vi "etc_XCITE_ExecuteCommand.vi"(8 "error in (no error)":errorcluster {"code" format="%x"}, 10 "command":string, 11 "h":u64) -> (0 "error out":errorcluster {"code" format="%x"}, 1 "answer":string, 2 "ErrorMessage":i32 format="%x", 3 "h out":u64)   [LabVIEW 2019, in "XCite.lvlib"]
doc: "Sends a command to execute on the slelected X-cite device."
uses:
  XCite.lvlib
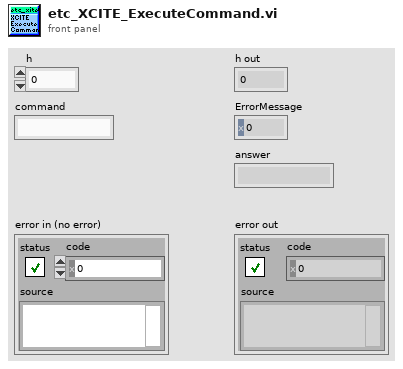
[diagram p1: front panel]
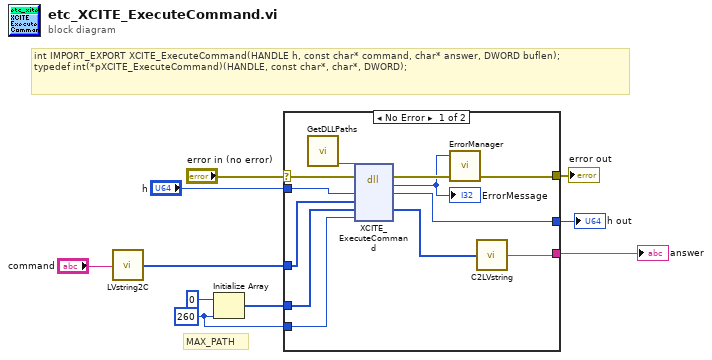
[diagram p0: block diagram]
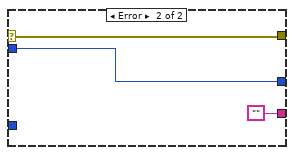
[diagram p2: hidden frame]
diagram:
  w3 = u16 260 ("dimension size")
  # "MAX_PATH"
  # "int IMPORT_EXPORT XCITE_ExecuteCommand(HANDLE h, const char* command, char* answer, DWORD buflen);\ntypedef int(*pXCITE_ExecuteCommand)(HANDLE, const char*, char*, DWORD);"
  n1 = call "LVstring2C.vi"("LVString"="command") -> ("CString"=w1:u8[])  [unwired: 3 in, 1 out]
  n2 = Initialize Array(u8 0, w3) -> (w4:u8[])
  n3 = case shown="No Error" "error in (no error)" {
    selector: "error in (no error)" -> [w22 w25]
    tunnel: [w20 w25] -> w10
    tunnel: "h" -> [w18 w24]
    tunnel: [w17 w24] -> w8
    tunnel: [w11 ""] -> w6
    tunnel: w1 -> [w15 _]
    tunnel: w4 -> [w14 _]
    tunnel: w3 -> [w13 _]
    frame No Error {
      n4 = call "GetDLLPaths.vi"() -> ("etc_xcite_path"=w16:path)  [unwired: 8 in, 3 out]
      n5 = dll-call lib="C:/LabVIEWDevFall2024/pco.labview/labview_sdk/runtime/bin64/etc_xcite.dll" fn="XCITE_ExecuteCommand"(path in=w16, error in=w22, "h"=w18, "command"=w15, "answer"=w14, "buflen"=w13) -> (error out=w21:errorcluster, "return type"=w19:i32, "h"=w17:u64, "answer"=w12:u8[])  [unwired: 3 in, 1 out]
      "ErrorMessage" <- w19
      n6 = call "ErrorManager.vi"("error in (no error)"=w21, "error code"=w19) -> ("error out"=w20:errorcluster)  [unwired: 2 in, 1 out]
      n7 = call "C2LVstring.vi"("CString"=w12) -> ("LVString"=w11:string)  [unwired: 4 in]
    }
    frame Error {
    }
  }
  "error out" <- w10
  "h out" <- w8
  "answer" <- w6
